vi "Actor Core.vi"(8 "error in":errorcluster, 11 "CS++IEFWerner in":refnum<class "CS++IEFWerner.lvclass">) -> (0 "error out":errorcluster, 3 "Actor out":refnum<class "Actor.lvclass">)   [LabVIEW 2015, in "CS++IEFWerner.lvlib" / "CS++IEFWerner.lvclass"]
doc: "(<B>Filename</B>: Actor Framework.lvlib:Actor.lvclass:Actor Core.vi)\n\nReceives messages to the actor, reacts to them, and initiates any error handling that may shut the actor down.\n\nDescendant classes may override this VI to append parallel tasks for the actor to complete while it handles messages. Overrides use the Call Parent Method node."
uses:
  CS++IEFWerner.lvclass
  <vilib>/ActorFramework/Actor/Actor.lvclass
  CS++IEFWerner.lvclass/CS++IEFWerner.ctl
  <vilib>/event_ctls.llb/usereventprio.ctl
  <vilib>/ActorFramework/Actor/Actor.lvclass/Actor.ctl
  <vilib>/ActorFramework/Message Enqueuer/Message Enqueuer.lvclass/Message Enqueuer.ctl
  <vilib>/ActorFramework/Report Error Msg/Report Error Msg.lvclass/Report Error Msg.ctl
  <vilib>/ActorFramework/Message Enqueuer/Enqueue.vi
  <vilib>/ActorFramework/Message Enqueuer/Init from Existing Queue.vi
  <vilib>/ActorFramework/Message Priority Queue/Priority Enqueue.vi
  CSPP_DeviceBase/CS++Motor/CS++Motor.lvclass
  <vilib>/ActorFramework/Report Error Msg/Report Error Msg.lvclass
  <vilib>/ActorFramework/Message Enqueuer/Message Enqueuer.lvclass
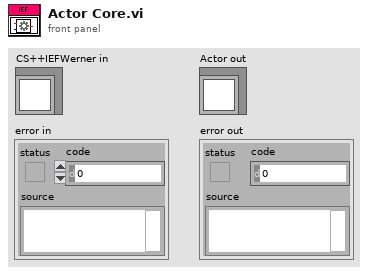
[diagram p1: front panel]
types:
  T1 = typedef "usereventprio.ctl" = enum32{"high priority", "normal priority"}
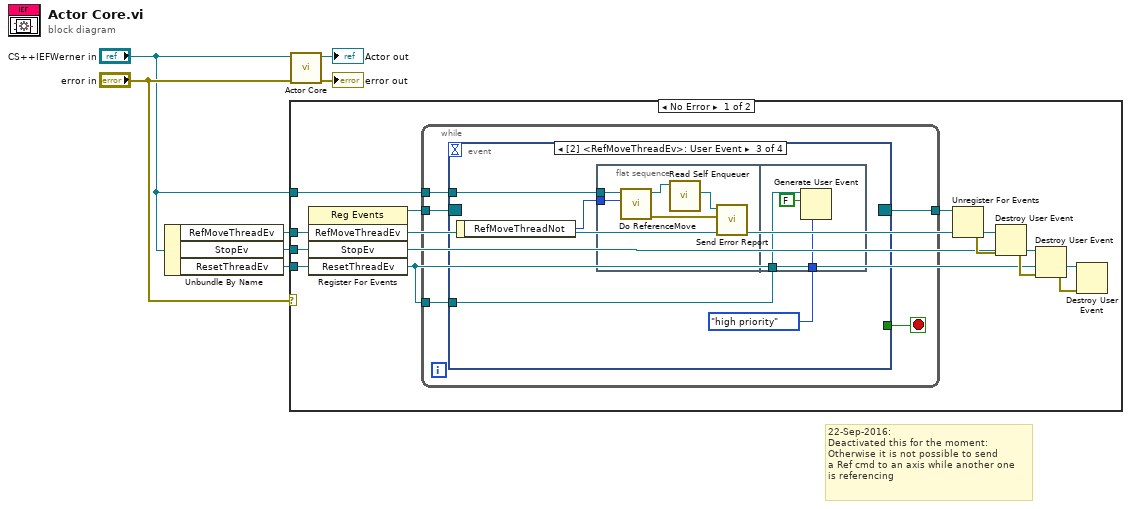
[diagram p0: block diagram]
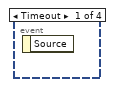
[diagram p2: hidden frame]
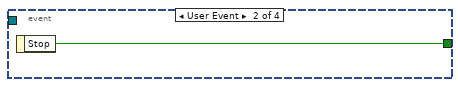
[diagram p3: hidden frame]
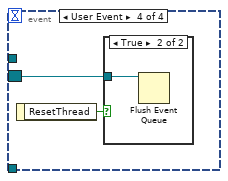
[diagram p4: hidden frame]
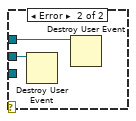
[diagram p6: hidden frame]
diagram:
  # "22-Sep-2016:\nDeactivated this for the moment:\nOtherwise it is not possible to send\na Ref cmd to an axis while another one\nis referencing"
  n1 = Unbundle By Name("CS++IEFWerner in") -> ("RefMoveThreadEv"=w4:refnum<user-event>, "StopEv"=w3:refnum<user-event>, "ResetThreadEv"=w1:refnum<user-event>)
  n2 = case shown="No Error" "error in" {
    tunnel: w4 -> [w13 w39]
    tunnel: w3 -> [w12 w38]
    tunnel: "CS++IEFWerner in" -> [w10 _]
    tunnel: w1 -> [w8 _]
    frame No Error {
      n3 = register-events(w13, w12, w8) -> (reference out=w16:refnum<event-registration>)  [unwired: 2 in, 1 out]
      n4 = while {
        tunnel: w16 -> [w21]
        tunnel: [w19] -> w15
        tunnel: w10 -> [w18]
        tunnel: w8 -> [w17]
        stop <- w20 stop-if-true
        n5 = event shown="[2] <RefMoveThreadEv>: User Event" {
          selector: w21 -> [_ _ _ w35]
          dyn-events: [_ _ _ _] -> w19
          timeout: _ -> [_ _ _ _]
          tunnel: [_ w22 _ _] -> w20
          tunnel: w18 -> [_ _ w26 _]
          tunnel: w17 -> [_ _ w24 _]
          event Timeout {
            n6 = event-data() -> ()  [unwired: 1 in, 1 out]
          }
          event User Event {
            n7 = event-data() -> ("Stop"=w22:bool)  [unwired: 1 in]
          }
          event User Event {
            n8 = event-data() -> ("RefMoveThreadNot"=w25:u16)  [unwired: 1 in]
            n9 = flat-sequence {
              tunnel: w26 -> [w31]
              tunnel: w25 -> [w30]
              tunnel: w24 -> [w34]
              tunnel: usereventprio."high priority" ("priority (normal)") -> [w32]
              frame #0 {
                n10 = call "Do ReferenceMove.vi"("AxisNumber"=w30, "CS++IEFWerner in"=w31) -> ("error out"=w29:errorcluster, "CS++IEFWerner out"=w28:refnum<class "CS++IEFWerner.lvclass">)  [unwired: 8 in]
                n11 = call <vilib>:"Read Self Enqueuer.vi"("Actor"=w28) -> ("Self Enqueuer"=w27:refnum<class "Message Enqueuer.lvclass">)  [unwired: 10 in]
                n12 = call <vilib>:"Send Error Report.vi"("Error From Sender"=w29, "Message Enqueuer"=w27) -> ()  [unwired: 9 in, 1 out]
              }
              frame #1 {
                n13 = Generate User Event(priority (normal)=w32, user event=w34, event data cluster=FALSE ("event data")) -> ()  [unwired: 1 in, 2 out]
              }
            }
          }
          event User Event {
            n14 = event-data() -> ("ResetThread"=w36:bool)  [unwired: 1 in]
            n15 = case shown="True" w36 {
              tunnel: w35 -> [_ w37]
              frame False {
              }
              frame True {
                n16 = Flush Event Queue(0:w37) -> ()  [unwired: 5 in, 3 out]
              }
            }
          }
        }
      }
      n17 = Unregister For Events(event registration refnum=w15) -> (error out=w14:errorcluster)  [unwired: 1 in]
      n18 = Destroy User Event(user event=w13, error in=w14) -> (error out=w11:errorcluster)
      n19 = Destroy User Event(user event=w12, error in=w11) -> (error out=w9:errorcluster)
      n20 = Destroy User Event(user event=w8, error in=w9) -> ()  [unwired: 1 out]
    }
    frame Error {
      n21 = Destroy User Event(user event=w38) -> ()  [unwired: 1 in, 1 out]
      n22 = Destroy User Event(user event=w39) -> ()  [unwired: 1 in, 1 out]
    }
  }
  n23 = call-parent "Actor Core.vi"("error in"="error in", "CS++BaseActor in"="CS++IEFWerner in") -> ("error out"=→"error out":errorcluster, "Actor out"=→"Actor out":refnum<class "Actor.lvclass">)  [unwired: 8 in]
